vi "basic - Read BSP Version.vi"() -> ()   [LabVIEW 2020]
uses:
  src/AIM664LV.lvlib
  src/_polimorphicInstances/session/Fdx Create Session (Generic-Board).vi
  src/_polimorphicInstances/session/Fdx Close Session (Board).vi
panel:
  out "BSP Version Parameters":string[][](table)
  out "BSP Special Version Out":T1
  out "BSP Version Out":T2
  in  "board":u32
  # "ARINC 664 Version"
  # "Overview: It helps to obtain the versions stored in the board.\n\nRequirement: One AIM ARINC-664 board with installed AIM ARINC 664 BSP.\nRestrictions: None.\nInstruction:\n1. Select the Board ID (0 if you have only one board in your system) and the port number. If you want to validate between two ports in one device, you can use tx board and Rx Boardd\n2. Run the VI.\n3. See the result in Current IRIG Time"
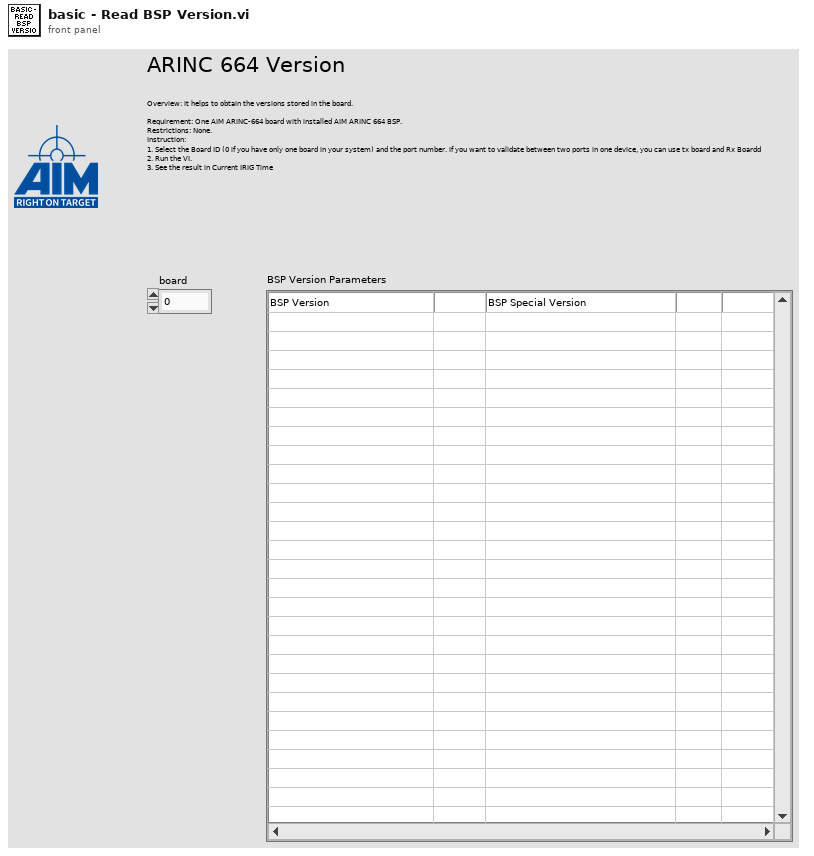
[diagram p1: front panel]
types:
  T1 = cluster{"SysDrvMajorSpecialVer":u32, "SysDrvMinorSpecialVer":u32, "DllMajorSpecialVer":u32, "DllMinorSpecialVer":u32, "TargetMajorSpecialVer":u32, "TargetMinorSpecialVer":u32, "FirmwareBiu1MajorSpecialVer":u32, "FirmwareBiu1MinorSpecialVer":u32, "FirmwareBiu2MajorSpecialVer":u32, "FirmwareBiu2MinorSpecialVer":u32, "MainLcaBuildNr":u32, "MainLcaMajorSpecialVer":u32, "MainLcaMinorSpecialVer":u32, "LcaBiu1BuildNr":u32, "LcaBiu1MajorSpecialVer":u32, "LcaBiu1MinorSpecialVer":u32, "LcaBiu2BuildNr":u32, "LcaBiu2MajorSpecialVer":u32, "LcaBiu2MinorSpecialVer":u32, "PciLcaBuildNr":u32, "PciLcaMajorSpecialVer":u32, "PciLcaMinorSpecialVer":u32, "TcpBuildNr":u32, "TcpMajorSpecialVer":u32, "TcpMinorSpecialVer":u32, "BootstrapMajorSpecialVer":u32, "BootstrapMinorSpecialVer":u32, "MonitorMajorSpecialVer":u32, "MonitorMinorSpecialVer":u32, "TargetOSMajorSpecialVer":u32, "TargetOSMinorSpecialVer":u32, "BspCompatibility":u32}
  T2 = cluster{"SysDrvMajorVer":u32, "SysDrvMinorVer":u32, "SysDrvBuildNr":u32, "DllMajorVer":u32, "DllMinorVer":u32, "DllBuildNr":u32, "TargetMajorVer":u32, "TargetMinorVer":u32, "TargetBuildNr":u32, "FirmwareBiu1MajorVer":u32, "FirmwareBiu1MinorVer":u32, "FirmwareBiu1BuildNr":u32, "FirmwareBiu2MajorVer":u32, "FirmwareBiu2MinorVer":u32, "FirmwareBiu2BuildNr":u32, "MainLcaMajorVer":u32, "MainLcaMinorVer":u32, "MainLcaBuildNr":u32, "LcaBiu1MajorVer":u32, "LcaBiu1MinorVer":u32, "LcaBiu2MajorVer":u32, "LcaBiu2MinorVer":u32, "PciLcaMajorVer":u32, "PciLcaMinorVer":u32, "TcpMajorVer":u32, "TcpMinorVer":u32, "BootstrapMajorVer":u32, "BootstrapMinorVer":u32, "MonitorMajorVer":u32, "MonitorMinorVer":u32, "TargetOSMajor":u32, "TargetOSMinor":u32, "BspCompatibility":u32}
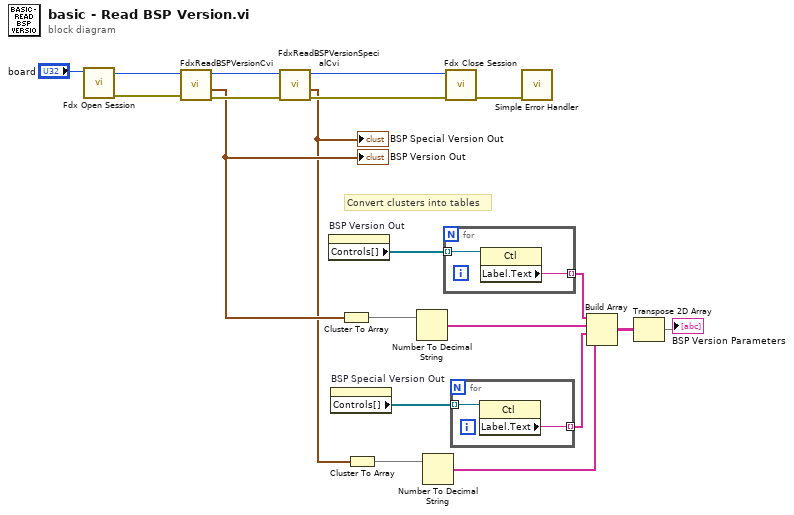
[diagram p0: block diagram]
diagram:
  # "Convert clusters into tables"
  n1 = call-poly "Fdx Open Session.vi"("board"="board") -> ("error out"=w20:errorcluster, "InstrumentHandle_board out"=w19:u32)  [unwired: 8 in, 1 out]
  n2 = call "FdxReadBSPVersionCvi.vi"("error in"=w20, "InstrumentHandle_board in"=w19) -> ("error out"=w17:errorcluster, "BSP Version Out"=w13:T2, "InstrumentHandle_board out"=w18:u32)  [unwired: 7 in]
  "BSP Version Out" <- w13
  n3 = call "FdxReadBSPVersionSpecialCvi.vi"("error in"=w17, "InstrumentHandle_board in"=w18) -> ("error out"=w16:errorcluster, "BSP Special Version Out"=w2:T1, "InstrumentHandle_board out"=w14:u32)  [unwired: 7 in]
  "BSP Special Version Out" <- w2
  n4 = property on="BSP Version Out" class="Clust (strict)"() -> ("Controls[]"=w8:refnum<vi>[])  [unwired: 2 in, 2 out]
  n5 = property on="BSP Special Version Out" class="Clust (strict)"() -> ("Controls[]"=w6:refnum<vi>[])  [unwired: 2 in, 2 out]
  n6 = Cluster To Array(cluster=w13) -> (array=w12:u32[])
  n7 = Cluster To Array(cluster=w2) -> (array=w3:u32[])
  n8 = Number To Decimal String(number=w12) -> (decimal integer string=w11:string[])  [unwired: 1 in]
  n9 = Number To Decimal String(number=w3) -> (decimal integer string=w1:string[])  [unwired: 1 in]
  n10 = for {
    tunnel: w8 -> [w22] mode=indexing
    tunnel: [w21] -> w7 mode=indexing
    n11 = property class="Ctl"(reference=w22) -> ("Label.Text"=w21:string)  [unwired: 1 in, 2 out]
  }
  n12 = call-poly "Fdx Close Session.vi"("error in (no error)"=w16, "InstrumentHandle_board in"=w14) -> ("error out"=w5:errorcluster)  [unwired: 9 in]
  n13 = for {
    tunnel: w6 -> [w24] mode=indexing
    tunnel: [w23] -> w4 mode=indexing
    n14 = property class="Ctl"(reference=w24) -> ("Label.Text"=w23:string)  [unwired: 1 in, 2 out]
  }
  n15 = call <vilib>:"Simple Error Handler.vi"("error in (no error)"=w5) -> ()  [unwired: 4 in, 5 out]
  n16 = Build Array(w7, w11, w4, w1) -> (w10:string[][])
  n17 = Transpose 2D Array(2D array=w10) -> (transposed array=→"BSP Version Parameters":string[][])
